vi "data to acc_gyro_enc.vi"(1 "gyro range (deg/s)":dbl=250.0, 2 "accel range (m/s2)":dbl=8.0, 3 "counts per rev":dbl=2048.0, 7 "byte array":u8[](array[numeric])) -> (8 "acc gyro data":T1)   [LabVIEW 2013]
uses:
  acc_gyro_enc_data.ctl
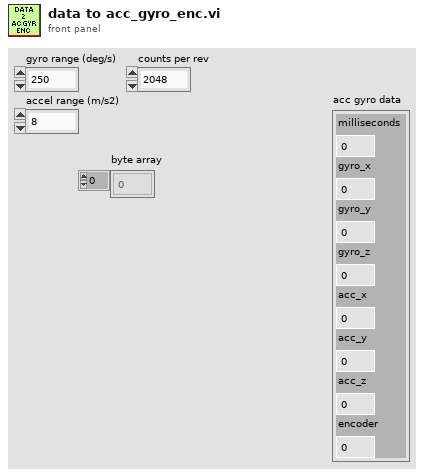
[diagram p1: front panel]
types:
  T1 = typedef "acc_gyro_enc_data.ctl" = cluster{"milliseconds":u64, "gyro_x":dbl, "gyro_y":dbl, "gyro_z":dbl, "acc_x":dbl, "acc_y":dbl, "acc_z":dbl, "encoder":dbl}
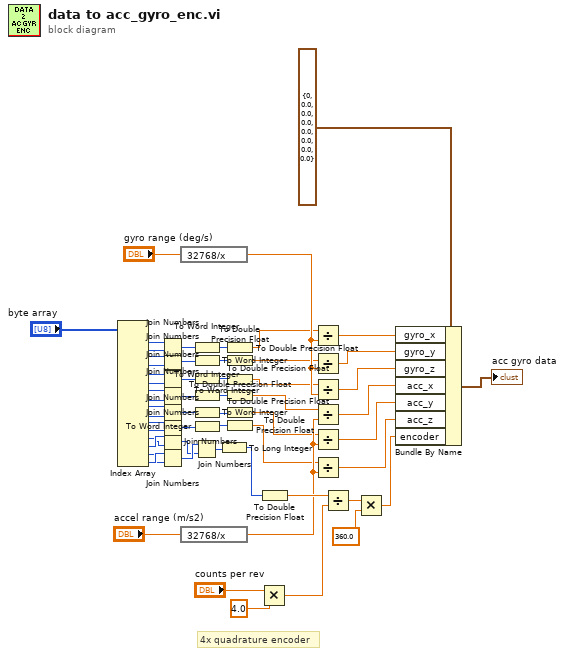
[diagram p0: block diagram]
diagram:
  # "4x quadrature encoder"
  n1 = Index Array(array="byte array") -> (element #1=w57:u8, element #2=w56:u8, element #3=w55:u8, element #4=w54:u8, element #5=w53:u8, element #6=w52:u8, element #7=w51:u8, element #8=w50:u8, element #9=w49:u8, element #10=w48:u8, element #11=w47:u8, element #12=w46:u8, element #13=w21:u8, element #14=w22:u8, element #15=w23:u8, element #16=w24:u8)  [unwired: 16 in]
  n2 = Join Numbers(hi=w57, lo=w56) -> ((hi.lo)=w45:u16)
  n3 = Join Numbers(hi=w55, lo=w54) -> ((hi.lo)=w44:u16)
  n4 = Join Numbers(hi=w53, lo=w52) -> ((hi.lo)=w43:u16)
  n5 = Join Numbers(hi=w51, lo=w50) -> ((hi.lo)=w42:u16)
  n6 = Join Numbers(hi=w49, lo=w48) -> ((hi.lo)=w41:u16)
  n7 = Join Numbers(hi=w47, lo=w46) -> ((hi.lo)=w40:u16)
  n8 = Join Numbers(hi=w22, lo=w21) -> ((hi.lo)=w19:u16)
  n9 = Join Numbers(hi=w24, lo=w23) -> ((hi.lo)=w20:u16)
  n10 = expression code="32768/x"("gyro range (deg/s)") -> (w9:dbl)
  n11 = expression code="32768/x"("accel range (m/s2)") -> (w4:dbl)
  n12 = To Word Integer(number=w45) -> (16bit integer=w39:i16)
  n13 = To Word Integer(number=w44) -> (16bit integer=w38:i16)
  n14 = To Word Integer(number=w43) -> (16bit integer=w37:i16)
  n15 = To Word Integer(number=w42) -> (16bit integer=w36:i16)
  n16 = To Word Integer(number=w41) -> (16bit integer=w35:i16)
  n17 = To Word Integer(number=w40) -> (16bit integer=w34:i16)
  n18 = Join Numbers(hi=w20, lo=w19) -> ((hi.lo)=w25:u32)
  n19 = To Long Integer(number=w25) -> (32bit integer=w18:i32)
  n20 = To Double Precision Float(number=w39) -> (double precision float=w8:dbl)
  n21 = To Double Precision Float(number=w38) -> (double precision float=w7:dbl)
  n22 = To Double Precision Float(number=w37) -> (double precision float=w6:dbl)
  n23 = To Double Precision Float(number=w36) -> (double precision float=w3:dbl)
  n24 = To Double Precision Float(number=w35) -> (double precision float=w2:dbl)
  n25 = To Double Precision Float(number=w34) -> (double precision float=w1:dbl)
  n26 = Multiply(x="counts per rev", y=4.0) -> (x*y=w15:dbl)
  n27 = To Double Precision Float(number=w18) -> (double precision float=w13:dbl)
  n28 = Divide(x=w8, y=w9) -> (x/y=w33:dbl)
  n29 = Divide(x=w7, y=w9) -> (x/y=w32:dbl)
  n30 = Divide(x=w6, y=w9) -> (x/y=w31:dbl)
  n31 = Divide(x=w3, y=w4) -> (x/y=w30:dbl)
  n32 = Divide(x=w2, y=w4) -> (x/y=w29:dbl)
  n33 = Divide(x=w1, y=w4) -> (x/y=w28:dbl)
  n34 = Divide(x=w13, y=w15) -> (x/y=w14:dbl)
  n35 = Multiply(x=w14, y=360.0) -> (x*y=w12:dbl)
  n36 = Bundle By Name(cluster=T1 {"milliseconds"=0, "gyro_x"=0.0, "gyro_y"=0.0, "gyro_z"=0.0, "acc_x"=0.0, "acc_y"=0.0, "acc_z"=0.0, "encoder"=0.0} ("acc gyro data"), "gyro_x"=w33, "gyro_y"=w32, "gyro_z"=w31, "acc_x"=w30, "acc_y"=w29, "acc_z"=w28, "encoder"=w12) -> (→"acc gyro data":T1)
